vi "Exercise9.4-FM_USRP_RX.vi"() -> ()   [LabVIEW 2013]
uses:
  <vilib>/sound2/lvsound2.llb/Sound Data Format.ctl
  <instrlib>/niUSRP/niUSRP Fetch Rx Data (CDB WDT).vi
  <vilib>/Analysis/2dsp.llb/Rational Resample (single channel, DBL).vi
  <vilib>/sound2/lvsound2.llb/Sound Output Write (DBL Single).vi
  <vilib>/express/express analysis/Spectral/Block/exnSpectralBlock spectral measurements RMS poly.vi
  <vilib>/express/express analysis/Spectral/Block/exnSpectralBlock spectral measurements RMS WFM.vi
  <vilib>/express/express analysis/Spectral/XNode/ExpressSpectralMeasurementsBlockNode.xnode
  <vilib>/Analysis/NI_AALPro.lvlib
panel:
  out "Spectrum (FFT)":cluster{"f0":dbl, "df":dbl, "magnitude":dbl[]}(graph)
  out "XY Graph":cluster{dbl[], dbl[]}(graph)
  out "error out":errorcluster
  in  "number of samples":i64=44100
  in  "sound format":T1={"sample rate (S/s)"=44100.0, "number of channels"=1, "bits per sample"=16}
  in  "stop":bool
  in  "active antenna":string="RX2"
  out "coerced gain":dbl=10.0 format="%#_6f"
  out "coerced carrier frequency":dbl=2400000000.0 format="%#_6p"
  out "coerced IQ rate":dbl=200000.0 format="%#_6p"
  in  "gain":dbl format="%#_6f"
  in  "carrier frequency":dbl=2400000000.0 format="%#_6p"
  in  "IQ rate":dbl=200000.0 format="%#_6p"
  in  "device names":refnum<k15>="192.168.10.2"
  out "error out":errorcluster
  # "FM Receiver"
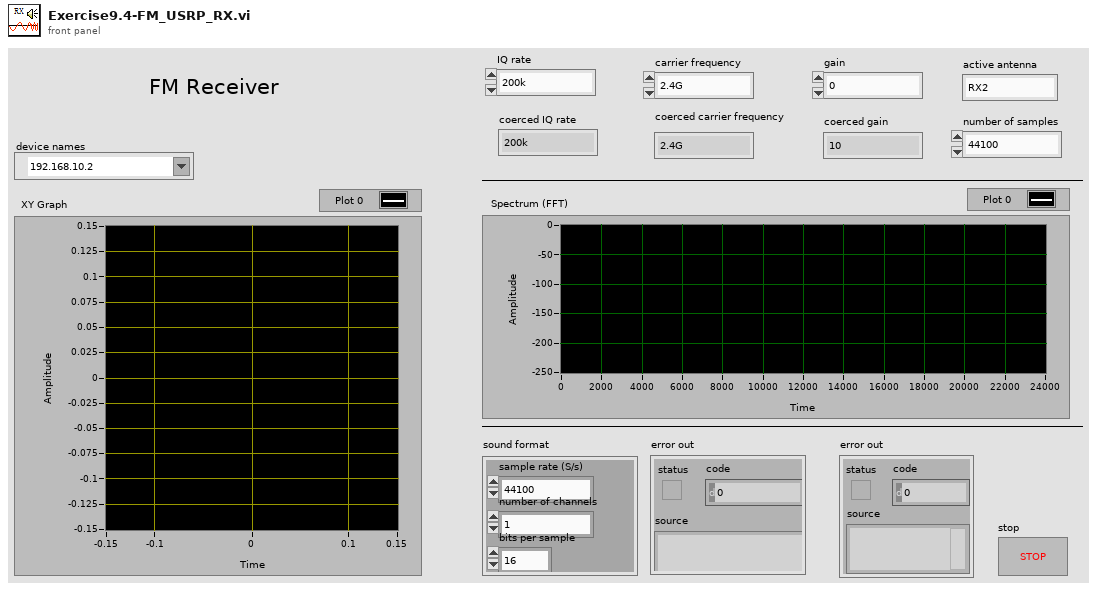
[diagram p1: front panel]
types:
  T1 = typedef "Sound Data Format.ctl" = cluster{"sample rate (S/s)":dbl, "number of channels":i32, "bits per sample":i32}
  T2 = typedef "Sound Output Task ID.ctl" = u32
  T3 = cluster{"averaging mode":u16, "weighting mode":u16, "number of averages":u32}
  T4 = cluster{"dB On (F)":bool, "unwrap phase (F)":bool, "convert to degree (F)":bool}
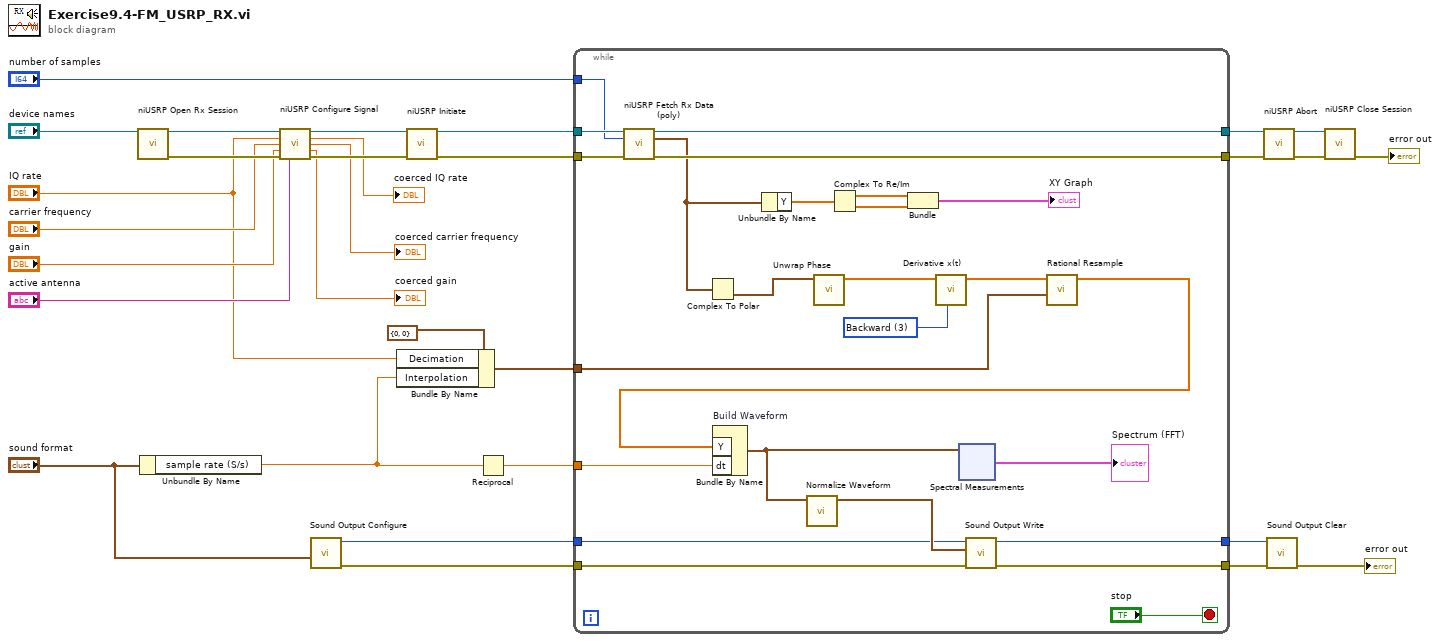
[diagram p0: block diagram]
diagram:
  n1 = call <instrlib>:"niUSRP Open Rx Session.vi"("device names"="device names") -> ("session handle out"=w29:refnum<k15>, "error out"=w28:errorcluster)  [unwired: 13 in]
  n2 = Unbundle By Name("sound format") -> ("sample rate (S/s)"=w4:dbl)
  n3 = call <instrlib>:"niUSRP Configure Signal.vi"("session handle"=w29, "IQ rate"="IQ rate", "carrier frequency"="carrier frequency", "gain"="gain", "error in (no error)"=w28, "active antenna"="active antenna") -> ("session handle out"=w19:refnum<k15>, "coerced IQ rate"=→"coerced IQ rate":dbl, "coerced carrier frequency"=→"coerced carrier frequency":dbl, "coerced gain"=→"coerced gain":dbl, "error out"=w21:errorcluster)  [unwired: 5 in]
  n4 = call <vilib>:"Sound Output Configure.vi"("sound format"="sound format") -> ("error out"=w14:errorcluster, "task ID"=w13:T2)  [unwired: 9 in]
  n5 = Bundle By Name(cluster=cluster{"Interpolation":i32, "Decimation":i32} {"Interpolation"=0, "Decimation"=0}, "Decimation"="IQ rate", "Interpolation"=w4) -> (w6:cluster{"Interpolation":i32, "Decimation":i32})
  n6 = call <instrlib>:"niUSRP Initiate.vi"("session handle"=w19, "error in (no error)"=w21) -> ("session handle out"=w24:refnum<k15>, "error out"=w23:errorcluster)  [unwired: 12 in]
  n7 = Reciprocal(x=w4) -> (1/x=w7:dbl)
  n8 = while {
    tunnel: w24 -> [w55]
    tunnel: w23 -> [w54]
    tunnel: [w53] -> w15
    tunnel: [w51] -> w3
    tunnel: w13 -> [w41]
    tunnel: w14 -> [w40]
    tunnel: [w47] -> w10
    tunnel: [w48] -> w11
    tunnel: "number of samples" -> [w45]
    tunnel: w7 -> [w43]
    tunnel: w6 -> [w42]
    stop <- "stop" stop-if-true
    w52 = u16 3 items=["2nd Order Central", "4th Order Central", "Forward", "Backward"] ("method")
    n9 = call-poly <instrlib>:"niUSRP Fetch Rx Data (poly).vi"("session handle"=w55, "number of samples"=w45, "error in (no error)"=w54) -> ("session handle out"=w53:refnum<k15>, "data"=w36:waveform(cdb), "error out"=w51:errorcluster)  [unwired: 9 in, 1 out]
    n10 = Complex To Polar(r * e^(i*theta)=w36) -> (theta=w37:waveform(dbl))  [unwired: 1 out]
    n11 = Unbundle By Name(w36) -> ("Y"=w35:cdb[])
    n12 = call <vilib>:"Unwrap Phase.vi"("Phase"=w37) -> ("Unwrapped Phase"=w39:dbl[])  [unwired: 9 in, 1 out]
    n13 = Complex To Re/Im(x + iy=w35) -> (x=w34:dbl[], y=w33:dbl[])
    n14 = Bundle(w34, w33) -> (→"XY Graph":cluster{dbl[], dbl[]})  [unwired: 1 in]
    n15 = call <vilib>:"Derivative x(t).vi"("method"=w52, "X"=w39) -> ("dX/dt"=w50:dbl[])  [unwired: 8 in, 1 out]
    n16 = call-poly <vilib>:"Rational Resample.vi"("resample factor"=w42, "X"=w50) -> ("Y"=w38:dbl[])  [unwired: 7 in, 2 out]
    n17 = Bundle By Name "Build Waveform"("Y"=w38, "dt"=w43) -> (w46:waveform(dbl))  [unwired: 1 in]
    n18 = call <vilib>:"Normalize Waveform.vi"("waveform in"=w46) -> ("normalized waveform"=w49:waveform(dbl))  [unwired: 7 in, 3 out]
    n19 = xnode "Spectral Measurements"("Signals"=w46) -> ("FFT - (RMS)"=→"Spectrum (FFT)":cluster{"f0":dbl, "df":dbl, "magnitude":dbl[]})  [unwired: 1 in, 2 out]
    n20 = call-poly <vilib>:"Sound Output Write.vi"("error in (no error)"=w40, "data"=w49, "task ID"=w41) -> ("error out"=w47:errorcluster, "task ID out"=w48:T2)  [unwired: 7 in]
  }
  n21 = call <instrlib>:"niUSRP Abort.vi"("session handle"=w15, "error in (no error)"=w3) -> ("session handle out"=w26:refnum<k15>, "error out"=w25:errorcluster)  [unwired: 12 in]
  n22 = call <vilib>:"Sound Output Clear.vi"("error in (no error)"=w10, "task ID"=w11) -> ("error out"=→"error out":errorcluster)  [unwired: 9 in]
  n23 = call <instrlib>:"niUSRP Close Session.vi"("session handle"=w26, "error in (no error)"=w25) -> ("error out"=→"error out":errorcluster)  [unwired: 13 in]
